vi "SMSD_position_pack.vi"(11 "DATA":u16[](array[numeric])) -> (3 "position":u32)   [LabVIEW 2019, in "SMSD.lvclass"]
uses:
  SMSD.lvclass
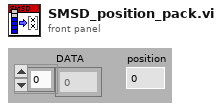
[diagram p1: front panel]
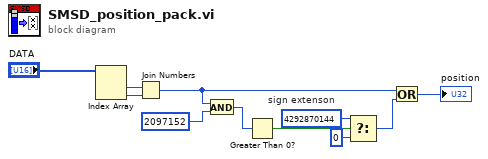
[diagram p0: block diagram]
diagram:
  w6 = u32 4292870144  # sign extenson
  n1 = Index Array(array="DATA") -> (element #1=w11:u16, element #2=w10:u16)  [unwired: 2 in]
  n2 = Join Numbers(hi=w11, lo=w10) -> ((hi.lo)=w2:u32)
  n3 = And(x=w2, y=u32 2097152) -> (x .and. y?=w8:u32)
  n4 = Greater Than 0?(x=w8) -> (x > 0?=w7:bool)
  n5 = Select(t=w6, s=w7, f=u32 0) -> (s? t:f=w4:u32)
  n6 = Or(x=w2, y=w4) -> (x .or. y?=→"position":u32)
